vi "SysDef.Property.Get.U32.Array.vi"(8 "error in (no error)":errorcluster, 9 "Value":u32[](array[numeric]), 10 "Property Name":string, 11 "nodeID":u64) -> (0 "error out":errorcluster, 1 "Value":u32[](array[numeric]), 3 "nodeID out":u64, 4 "Found?":bool)   [LabVIEW 2019, in "Advanced System Definition.lvlib"]
uses:
  SysDef API/Advanced System Definition.lvlib
  <vilib>/NI VeriStand/Custom Device API/Get Item Property (U32 Array).vi
  NationalInstruments.VeriStand.SystemDefinitionAPI
  <vilib>/NI VeriStand/Custom Device API/Custom Device API.lvlib
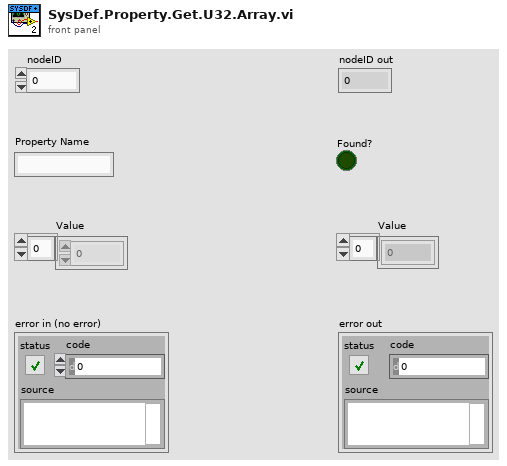
[diagram p1: front panel]
types:
  T1 = typedef "Custom Device API.lvlib/Custom Device Item Ref.ctl" = u64
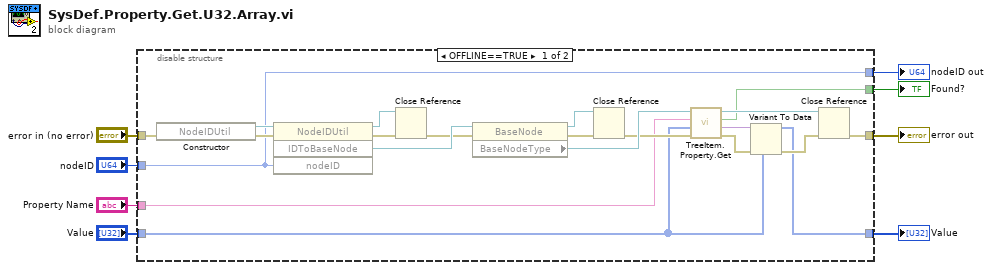
[diagram p0: block diagram]
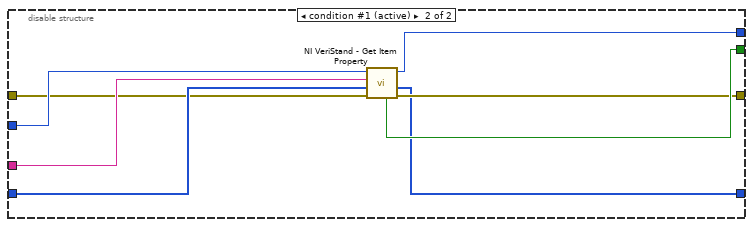
[diagram p2: hidden frame]
diagram:
  n1 = disable-structure shown="OFFLINE==TRUE" {
    disable-tunnel: "error in (no error)" -> [w22 w34]
    disable-tunnel: "nodeID" -> [w9 w35]
    disable-tunnel: [w17 w32] -> w6
    disable-tunnel: "Property Name" -> [w16 w36]
    disable-tunnel: [w12 w33] -> w4
    disable-tunnel: "Value" -> [w11 w37]
    disable-tunnel: [w10 w30] -> w2
    disable-tunnel: [w9 w31] -> w1
    frame condition #0 {
      n2 = constructor class="NodeIDUtil"(error in=w22) -> (reference out=w29:refnum<k24>, error out=w28:errorcluster)  [unwired: 2 in, 1 out]
      n3 = invoke class="NodeIDUtil" method="IDToBaseNode"(reference=w29, error in=w28, "nodeID"=w9) -> (reference out=w23:refnum<k24>, error out=w25:errorcluster, "IDToBaseNode"=w27:refnum<k24>)  [unwired: 1 in, 1 out]
      n4 = Close Reference(reference=w23, error in (no error)=w25) -> (error out=w24:errorcluster)
      n5 = property class="BaseNode"(reference=w27, error in=w24) -> (reference out=w21:refnum<k24>, error out=w20:errorcluster, "BaseNodeType"=w26:refnum<k24>)
      n6 = Close Reference(reference=w21, error in (no error)=w20) -> (error out=w19:errorcluster)
      n7 = call "TreeItem.Property.Get.vi"("error in (no error)"=w19, "Default Value"=w11, "Property Name"=w16, "Basenode"=w26) -> ("error out"=w14:errorcluster, "Variant"=w15:variant, "Found?"=w12:bool, "Basenode"=w18:refnum<k24>)  [unwired: 4 in]
      n8 = Variant To Data(error in=w14, type=w11, Variant=w15) -> (data=w10:u32[], error out=w13:errorcluster)
      n9 = Close Reference(reference=w18, error in (no error)=w13) -> (error out=w17:errorcluster)
    }
    frame condition #1 (active) {
      n10 = call-poly <vilib>:"NI VeriStand - Get Item Property.vi"("error in (no error)"=w34, "Default Value"=w37, "Property Name"=w36, "Item Ref in"=w35) -> ("error out"=w32:errorcluster, "Value"=w30:u32[], "Item Ref out"=w31:T1, "Found?"=w33:bool)  [unwired: 4 in]
    }
  }
  "nodeID out" <- w1
  "error out" <- w6
  "Value" <- w2
  "Found?" <- w4
